vi "VerticalTrajectory2.vi"(3 "speed 1":i32, 4 "step":dbl, 5 "z2":dbl, 6 "z1":dbl, 7 "x":dbl) -> ()   [LabVIEW 2018]
uses:
  ARM angles.vi
panel:
  out "old wr":i32
  out "e2":i32
  out "e1":i32
  out "qo1":i32
  out "qo2":i32
  out "wr":i32
  out "busy 2":bool
  out "busy 1":bool
  out "s2":i32
  out "s1":i32
  out "q2":dbl
  out "q1":dbl
  in  "dt":dbl
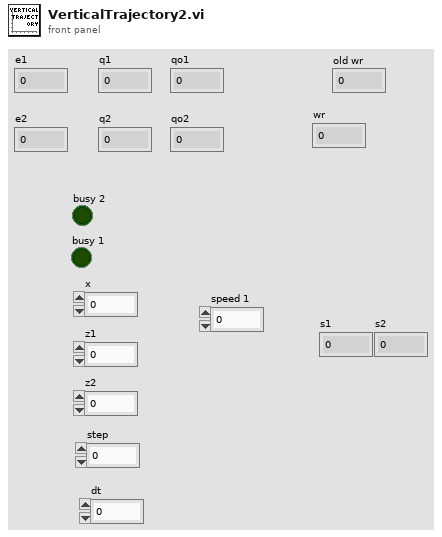
[diagram p1: front panel]
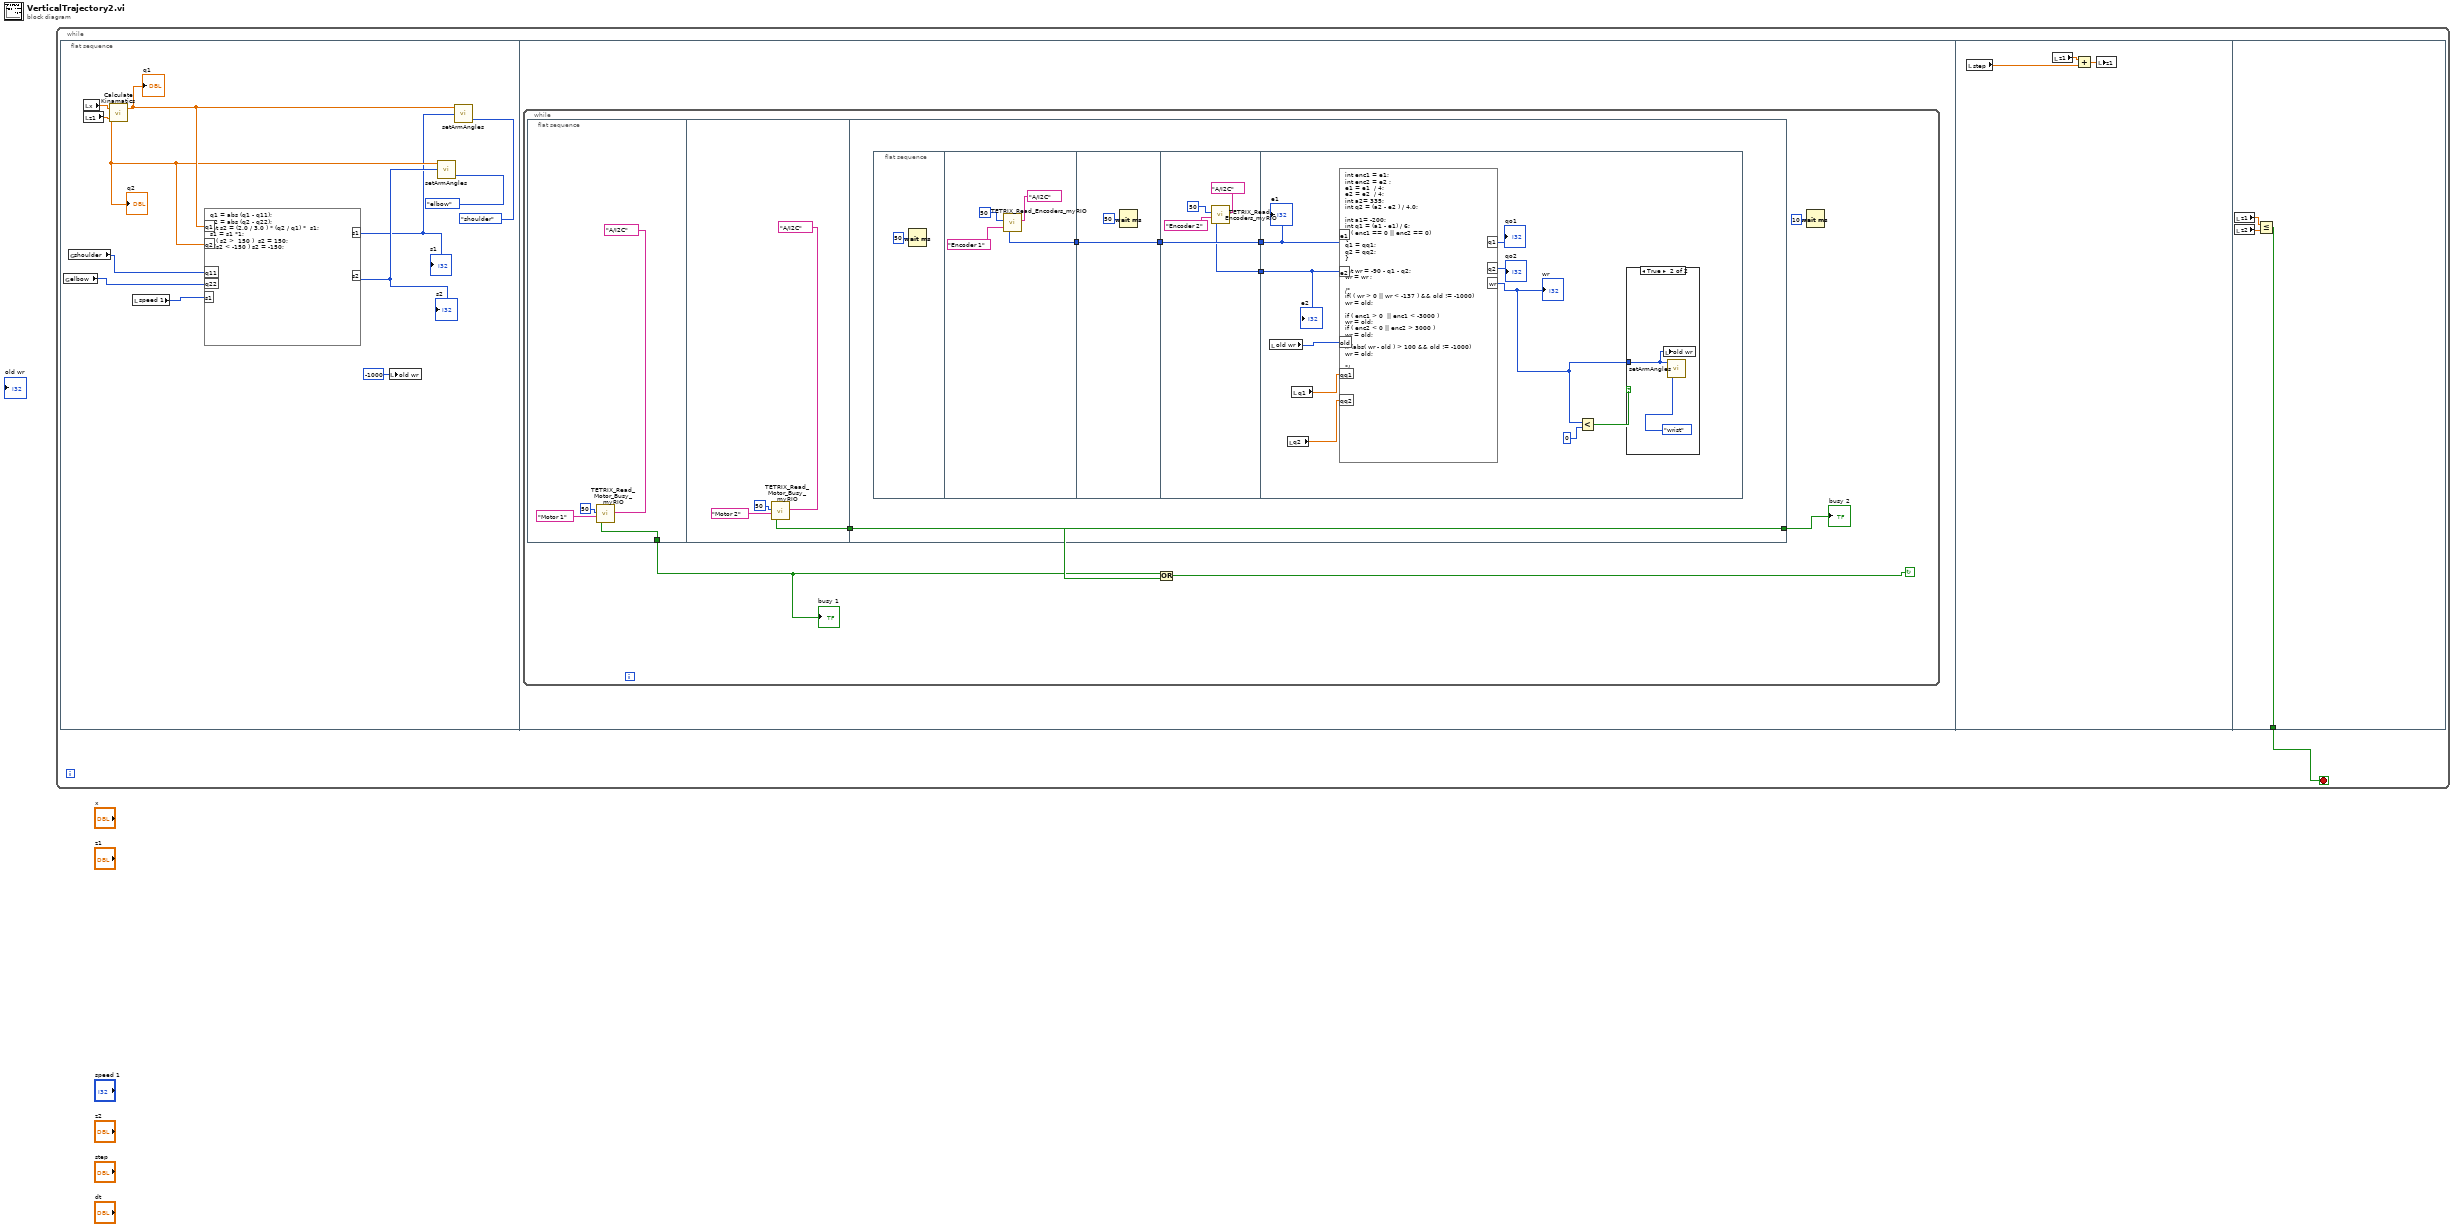
[diagram p0: block diagram]
diagram:
  n1 = while {
    stop <- w1 stop-if-true
    n2 = flat-sequence {
      tunnel: [w59] -> w1
      frame #0 {
        n3 = global read "ARM angles.vi" "elbow"() -> (w3:i32)
        n4 = global read "ARM angles.vi" "shoulder"() -> (w4:i32)
        n5 = local read "x"() -> (w13:dbl)
        n6 = local read "z1"() -> (w12:dbl)
        n7 = call "Calculate Kinamatics.vi"("y"=w12, "x"=w13) -> ("q2"=w8:dbl, "q1"=w9:dbl)
        "q2" <- w8
        "q1" <- w9
        n8 = local read "speed 1"() -> (w7:i32)
        n9 = formula code="q1 = abs (q1 - q11);\nq2 = abs (q2 - q22);\nint s2 = (2.0 / 3.0 ) * (q2 / q1) *  s1;\ns1 = s1 *1;\nif ( s2 >  150 )  s2 = 150;\nif(s2 < -150 ) s2 = -150;"("q1"=w9, "q2"=w8, "s1"=w7, "q11"=w4, "q22"=w3) -> ("s1"=w5:i32, "s2"=w6:i32)
        "s1" <- w5
        "s2" <- w6
        n10 = local write "old wr"(-1000 ("old wr")) -> ()
        n11 = call "setArmAngles.vi"("Enum"=enum16{"shoulder", "elbow", "wrist"}."elbow", "speed"=w6, "angle"=w8) -> ()  [unwired: 1 in]
        n12 = call "setArmAngles.vi"("Enum"=enum16{"shoulder", "elbow", "wrist"}."shoulder", "speed"=w5, "angle"=w9) -> ()  [unwired: 1 in]
      }
      frame #1 {
        n13 = while {
          stop <- w14 continue-if-true
          n14 = flat-sequence {
            tunnel: [w19] -> w17
            tunnel: [w23] -> w15
            tunnel: [w31] -> w18
            tunnel: w15 -> [w31]
            frame #0 {
              n15 = call <vilib>:"TETRIX_Read_Motor_Busy_myRIO.vi"("myRIO MXP Port A/B"=tag "A/I2C", "Select Channel"="Motor 1", "Controller ID#  (I2C Address)"=u8 50) -> ("Motor Busy?"=w19:bool)  [unwired: 3 in, 1 out]
            }
            frame #1 {
              n16 = call <vilib>:"TETRIX_Read_Motor_Busy_myRIO.vi"("myRIO MXP Port A/B"=tag "A/I2C", "Select Channel"="Motor 2", "Controller ID#  (I2C Address)"=u8 50) -> ("Motor Busy?"=w23:bool)  [unwired: 3 in, 1 out]
            }
            frame #2 {
              n17 = flat-sequence {
                tunnel: [w33] -> w28
                tunnel: w28 -> [w38]
                tunnel: [w38] -> w27
                tunnel: w27 -> [w40]
                tunnel: [w40] -> w30
                tunnel: [w39] -> w29
                tunnel: w30 -> [w53]
                tunnel: w29 -> [w52]
                frame #0 {
                  n18 = Wait (ms)(milliseconds to wait=u32 50) -> ()  [unwired: 1 out]
                }
                frame #1 {
                  n19 = call <vilib>:"TETRIX_Read_Encoders_myRIO.vi"("myRIO MXP Port A/B"=tag "A/I2C", "Select Encoder"="Encoder 1", "Controller ID#  (I2C Address)"=u8 50) -> ("Encoder Output"=w33:i32)  [unwired: 3 in, 1 out]
                }
                frame #2 {
                  n20 = Wait (ms)(milliseconds to wait=u32 50) -> ()  [unwired: 1 out]
                }
                frame #3 {
                  n21 = call <vilib>:"TETRIX_Read_Encoders_myRIO.vi"("myRIO MXP Port A/B"=tag "A/I2C", "Select Encoder"="Encoder 2", "Controller ID#  (I2C Address)"=u8 50) -> ("Encoder Output"=w39:i32)  [unwired: 3 in, 1 out]
                }
                frame #4 {
                  n22 = local read "old wr"() -> (w49:i32)
                  n23 = local read "q2"() -> (w47:dbl)
                  n24 = local read "q1"() -> (w48:dbl)
                  n25 = formula code="int enc1 = e1;\nint enc2 = e2 ;\ne1 = e1  / 4;\ne2 = e2  / 4;\nint a2= 335;\nint q2 = (a2 - e2 ) / 4.0;\n\nint a1= -200;\nint q1 = (a1 - e1) / 6;\nif ( enc1 == 0 || enc2 == 0)\n{\nq1 = qq1;\nq2 = qq2;\n}\n\nint wr = -90 - q1 - q2;\nwr = wr ;\n\n/*\nif( ( wr > 0 || wr < -137 ) && old != -1000)\nwr = old;\n\nif ( enc1 > 0  || enc1 < -3000 )\nwr = old;\nif ( enc2 < 0 || enc2 > 3000 )\nwr = old;\n\nif (abs( wr - old ) > 100 && old != -1000) \nwr = old;\n\n*/"("e1"=w53, "e2"=w52, "old"=w49, "qq1"=w48, "qq2"=w47) -> ("q1"=→"qo1":i32, "q2"=→"qo2":i32, "wr"=w44:i32)
                  "wr" <- w44
                  n26 = Less?(x=w44, y=0) -> (x < y?=w45:bool)
                  n27 = case shown="True" w45 {
                    tunnel: w44 -> [_ w54]
                    frame False {
                    }
                    frame True {
                      n28 = local write "old wr"(w54) -> ()
                      n29 = call "setArmAngles.vi"("Enum"=enum16{"shoulder", "elbow", "wrist"}."wrist", "angle"=w54) -> ()  [unwired: 2 in]
                    }
                  }
                  "e1" <- w53
                  "e2" <- w52
                }
              }
            }
          }
          n30 = Or(x=w17, y=w18) -> (x .or. y?=w14:bool)
          n31 = Wait (ms)(milliseconds to wait=u32 10) -> ()  [unwired: 1 out]
          "busy 2" <- w18
          "busy 1" <- w17
        }
      }
      frame #2 {
        n32 = local read "step"() -> (w57:dbl)
        n33 = local read "z1"() -> (w58:dbl)
        n34 = Add(x=w58, y=w57) -> (x+y=w56:dbl)
        n35 = local write "z1"(w56) -> ()
      }
      frame #3 {
        n36 = local read "z1"() -> (w60:dbl)
        n37 = local read "z2"() -> (w61:dbl)
        n38 = Less Or Equal?(x=w60, y=w61) -> (x <= y?=w59:bool)
      }
    }
  }
